vi "BenchmarkName.vi"() -> (1 "process name":string)   [LabVIEW 2017, in "Benchmarking.lvlib"]
uses:
  <vilib>/addons/InsightCM/Devices/Shared/Common/Benchmarking/Benchmarking.lvlib
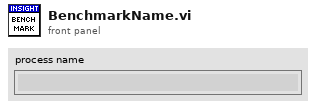
[diagram p1: front panel]
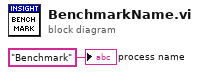
[diagram p0: block diagram]
diagram:
  "process name" <- "Benchmark" ("ProcessName")
